vi "Setup.vi"(11 "Queue Transport in":refnum<class "Queue Transport.lvclass">) -> (0 "Error out":errorcluster, 3 "Queue Transport out":refnum<class "Queue Transport.lvclass">)   [LabVIEW 2025, in "jettl.lvlib" / "Transport.lvlib" / "Queue Transport.lvclass"]
uses:
  Queue Transport.lvclass
  Msg/Msg.lvclass
  Queue Transport.lvclass/Queue Transport.ctl
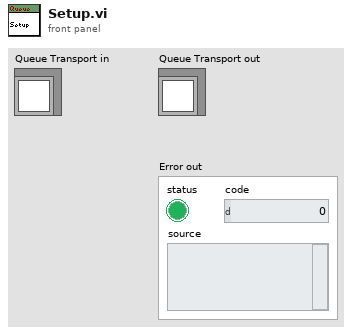
[diagram p1: front panel]
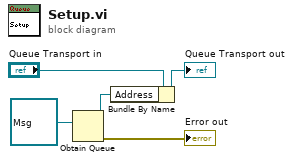
[diagram p0: block diagram]
diagram:
  n1 = Obtain Queue(element data type=refnum<class "Msg.lvclass"> refnum ("Msg")) -> (queue out=w2:refnum<queue>, error out=→"Error out":errorcluster)  [unwired: 4 in, 1 out]
  n2 = Bundle By Name(cluster="Queue Transport in", "Address"=w2) -> (→"Queue Transport out":refnum<class "Queue Transport.lvclass">)
